vi "ImageFixGrab.vi"(8 "error in (no error)":errorcluster, 11 "Image in":refnum<class "Image.lvclass">) -> (0 "error out":errorcluster, 3 "Image out":refnum<class "Image.lvclass">)   [LabVIEW 2012, in "Image.lvclass"]
uses:
  classes/Image.lvclass
  classes/Image.lvclass/Image.ctl
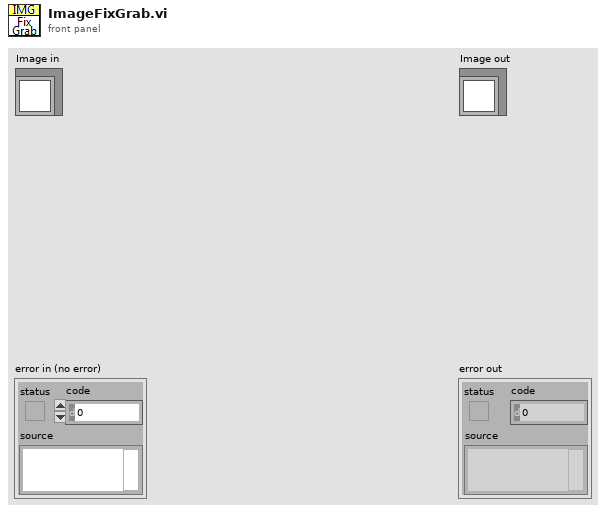
[diagram p1: front panel]
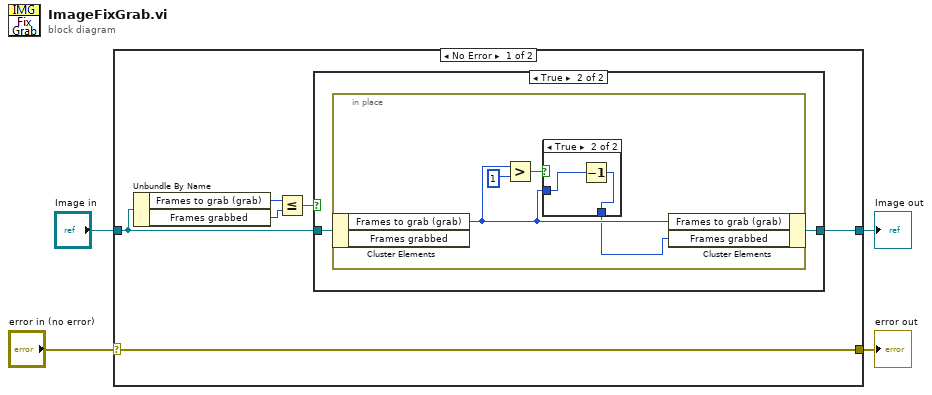
[diagram p0: block diagram]
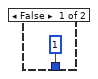
[diagram p3: hidden frame]
diagram:
  n1 = case shown="No Error" "error in (no error)" {
    selector: "error in (no error)" -> [w10 w22]
    tunnel: [w10 w22] -> w3
    tunnel: [w5 w21] -> w1
    tunnel: "Image in" -> [w6 w21]
    frame No Error {
      n2 = Unbundle By Name(w6) -> ("Frames to grab (grab)"=w9:i32, "Frames grabbed"=w8:i32)
      n3 = Less Or Equal?(x=w9, y=w8) -> (x <= y?=w7:bool)
      n4 = case shown="True" w7 {
        tunnel: w6 -> [w11 w13]
        tunnel: [w11 w12] -> w5
        frame False {
        }
        frame True {
          n5 = in-place {
            n6 = in-place-cluster #1(w13) -> ("Frames to grab (grab)"=w15:i32)  [unwired: 1 out]
            n7 = Greater?(x=w15, y=1) -> (0:w17:bool)
            n8 = case shown="True" w17 {
              tunnel: w15 -> [_ w20]
              tunnel: [1 w19] -> w14
              frame False {
              }
              frame True {
                n9 = Decrement(x=w20) -> (x-1=w19:i32)
              }
            }
            n10 = in-place-cluster #1("Frames to grab (grab)"=w15, "Frames grabbed"=w14) -> (w12:refnum<class "Image.lvclass">)
          }
        }
      }
    }
    frame Error {
    }
  }
  "error out" <- w3
  "Image out" <- w1
